vi "Write Com_Set.vi"(8 "error in (no error)":errorcluster, 10 "Com_Set":T1, 11 "Modbus In":refnum<class "Modbus.lvclass">) -> (0 "error out":errorcluster, 3 "Modbus Out":refnum<class "Modbus.lvclass">)   [LabVIEW 2019, in "Modbus.lvclass"]
uses:
  Modbus.lvclass
  SettingCtrl.ctl
  Modbus.lvclass/Modbus.ctl
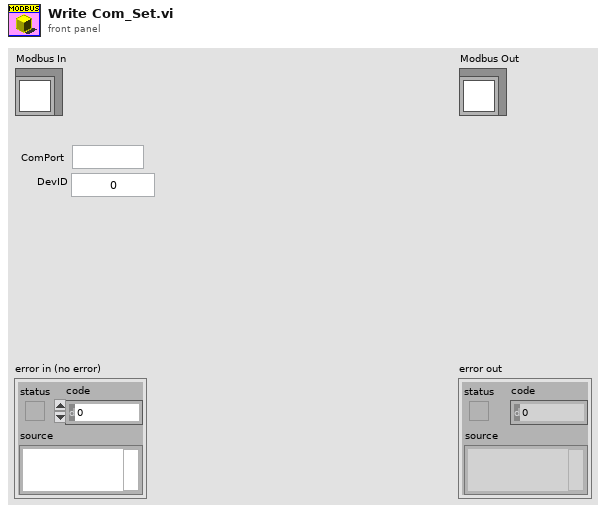
[diagram p1: front panel]
types:
  T1 = typedef "Modbus.lvclass/SettingCtrl.ctl" = cluster{"DevID":u16, "ComPort":string}
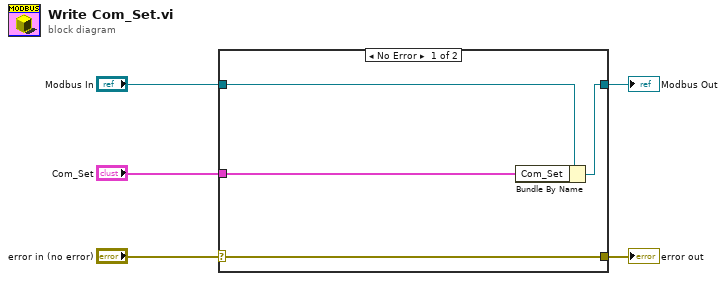
[diagram p0: block diagram]
diagram:
  n1 = case shown="No Error" "error in (no error)" {
    selector: "error in (no error)" -> [w9 w10]
    tunnel: [w9 w10] -> w4
    tunnel: [w7 w11] -> w2
    tunnel: "Modbus In" -> [w8 w11]
    tunnel: "Com_Set" -> [w6 _]
    frame No Error {
      n2 = Bundle By Name(cluster=w8, "Com_Set"=w6) -> (w7:refnum<class "Modbus.lvclass">)
    }
    frame Error {
    }
  }
  "error out" <- w4
  "Modbus Out" <- w2
